vi "Scatter-Gather Write Iterator.vi"(8 "error in (no error)":errorcluster, 9 "Iterations (1000)":i32=110, 10 "Channel Count":i32, 11 "GE 5565PIORC in":refnum<class "GE 5565PIORC Old.lvclass">) -> (0 "error out":errorcluster, 1 "Histogram Graph":T1(graph), 2 "Metrics":T2 {"Transfer Rate" format="%.2pB/s"; "Duration Std. Dev." format="%.0f µs"; "Duration Average" format="%.0f µs"}, 3 "GE 5565PIORC out":refnum<class "GE 5565PIORC Old.lvclass">)   [LabVIEW 2016]
uses:
  Source/GE 5565PIORC/GE 5565PIORC Old.lvclass
  Controls/Throughput Metrics.ctl
  Source/GE 5565PIORC/GE 5565PIORC Old.lvclass/GE 5565PIORC Old.ctl
  Source/GE 5565PIORC/VIs/Block Operations/Allocate Multiple Blocks.vi
  Source/GE 5565PIORC/VIs/DMA/DMA.Create Transfer (Multiple Blocks).vi
  Source/GE 5565PIORC/VIs/Block Operations/Allocate Single Block.vi
  Source/GE 5565PIORC/VIs/DMA/DMA.Transfer Size.vi
  Source/GE 5565PIORC/VIs/Registers/Local Configuration.PCI Address.Set.vi
  Source/GE 5565PIORC/VIs/Registers/Local Configuration.DMADPR0.First Descriptor Address.Set.vi
  Source/GE 5565PIORC/VIs/DMA/DMA.Scatter-Gather.Link Block Descriptors.vi
  Source/GE 5565PIORC/VIs/DMA/DMA.Scatter-Gather.Commit Blocks.vi
  Source/GE 5565PIORC/VIs/Registers/Local Configuration.Local Address.Set.vi
  Source/GE 5565PIORC/VIs/Registers/Local Configuration.Transfer Size.Set.vi
  Source/GE 5565PIORC/VIs/Registers/Local Configuration.DMADPR0.Transfer Direction.Set.vi
  Source/GE 5565PIORC/VIs/Registers/Local Configuration.DMAMODE0.Scatter-Gather Enable.Set.vi
  <vilib>/Utility/error.llb/Clear Errors.vi
  Source/GE 5565PIORC/VIs/Registers/Local Configuration.DMACSR0.DMA Start.Set.vi
  Source/GE 5565PIORC/VIs/Interrupts/Wait for PXI Interrupt Events.vi
  Source/GE 5565PIORC/VIs/Registers/Local Configuration.DMACSR0.DMA Clear Interrupt.Set.vi
  Source/GE 5565PIORC/VIs/Binary Operations/Align to 8-byte Boundary.vi
  Source/GE 5565PIORC/VIs/Binary Operations/Align to 16-byte Boundary.vi
  Source/GE 5565PIORC/VIs/Registers/Local Configuration.Get Register Offset.vi
  Source/GE 5565PIORC/VIs/Binary Operations/Set Bits.vi
  Source/GE 5565PIORC/VIs/Binary Operations/Set Bits U32.vi
  Source/GE 5565PIORC/VIs/Binary Operations/Get Bits.vi
  Source/GE 5565PIORC/VIs/Binary Operations/Get Bits U32.vi
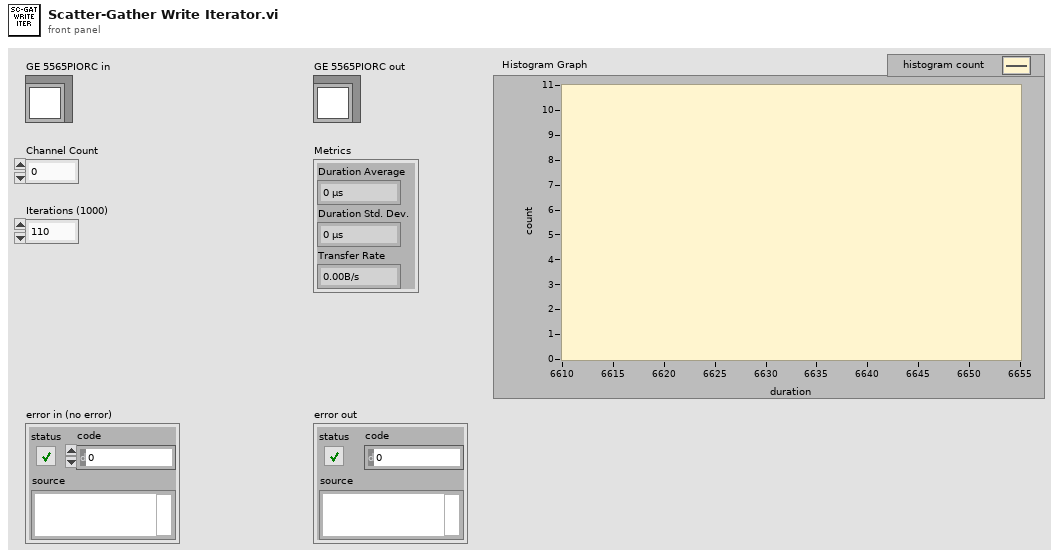
[diagram p1: front panel]
types:
  T1 = cluster{"X Values":dbl[], "Histogram: h(x)":i32[]}
  T2 = typedef "Throughput Metrics.ctl" = cluster{"Duration Average":u32, "Duration Std. Dev.":u32, "Transfer Rate":dbl}
  T3 = typedef "GE 5565PIORC Old.lvclass/DMA Block Descriptor.ctl" = cluster{"descriptor ptr (VISA)":u32, "descriptor size":u32, "descriptor ptr (aligned)":u32, "data ptr (lower)":u32, "data ptr (upper)":u32, "data size":u32, "next descriptor ptr":u32}
  T4 = typedef "GE 5565PIORC Old.lvclass/DMA Transfer Spec.ctl" = cluster{"RFM Address":u32, "Block Descriptors":T3[]}
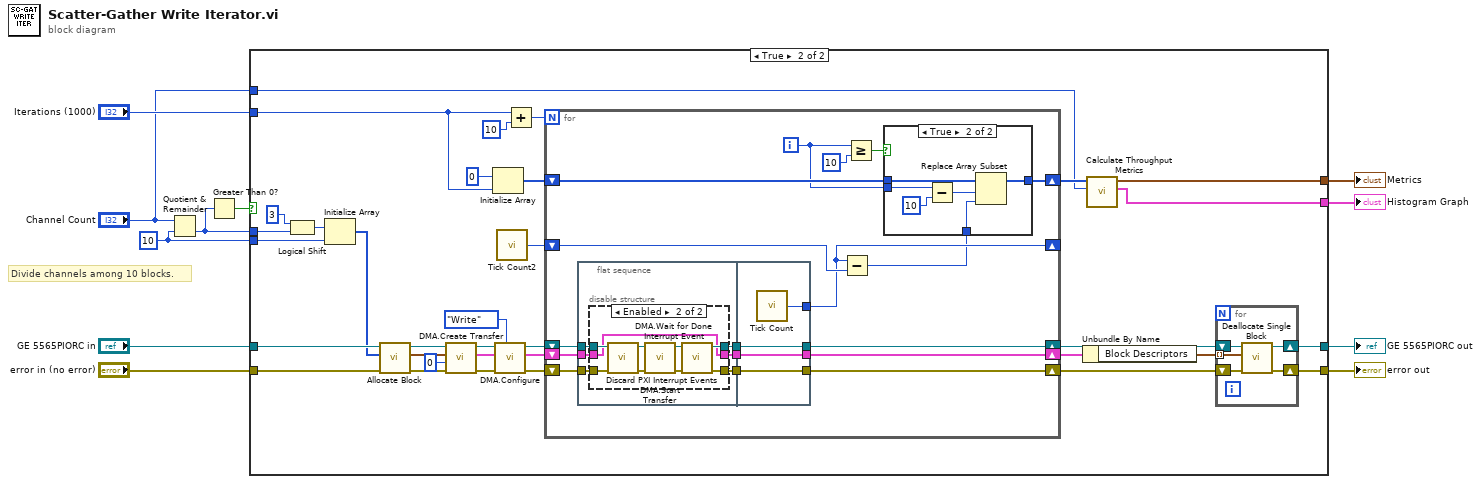
[diagram p0: block diagram]
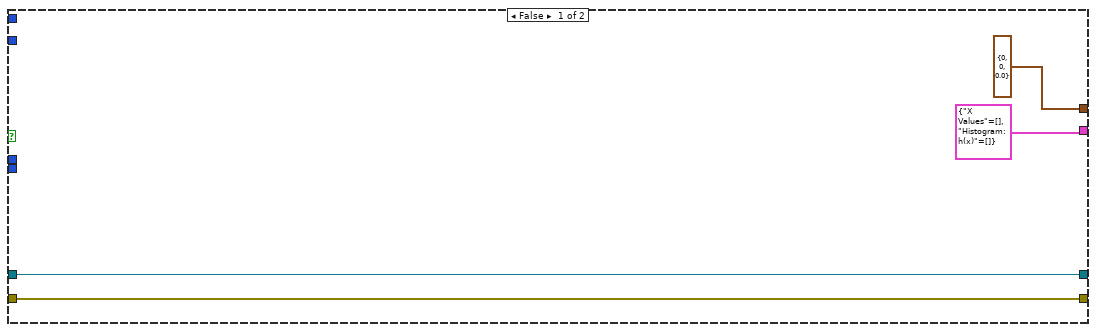
[diagram p2: hidden frame]
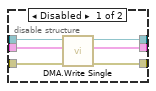
[diagram p4: hidden frame]
diagram:
  w4 = 10 ("y")
  # "Divide channels among 10 blocks."
  n1 = Quotient & Remainder(x="Channel Count", y=w4) -> (floor(x/y)=w2:i32)  [unwired: 1 out]
  n2 = Greater Than 0?(x=w2) -> (x > 0?=w1:bool)
  n3 = case shown="True" w1 {
    tunnel: [w15 w47] -> w11
    tunnel: [w12 w46] -> w10
    tunnel: "Iterations (1000)" -> [_ w40]
    tunnel: [T2 {"Duration Average"=0, "Duration Std. Dev."=0, "Transfer Rate"=0.0} ("Metrics") w36] -> w8
    tunnel: [T1 {"X Values"=[], "Histogram: h(x)"=[]} ("Histogram Graph") w35] -> w7
    tunnel: "GE 5565PIORC in" -> [w12 w34]
    tunnel: "error in (no error)" -> [w15 w33]
    tunnel: w4 -> [_ w29]
    tunnel: w2 -> [_ w28]
    tunnel: "Channel Count" -> [_ w25]
    frame False {
    }
    frame True {
      n4 = Logical Shift(y=i16 3, x=w28) -> (x << y=w27:i32)
      n5 = Initialize Array(w27, w29) -> (w23:i32[])
      n6 = call-poly "Allocate Block.vi"("error in (no error)"=w33, "sizes (bytes)"=w23, "GE 5565PIORC in"=w34) -> ("error out"=w31:errorcluster, "Block Descriptors"=w30:T3[], "GE 5565PIORC out"=w32:refnum<class "GE 5565PIORC Old.lvclass">)  [unwired: 6 in]
      n7 = call-poly "DMA.Create Transfer.vi"("error in (no error)"=w31, "RFM Offset"=u32 0, "Block Descriptors"=w30, "GE 5565PIORC in"=w32) -> ("error out"=w20:errorcluster, "DMA Transfer Spec"=w19:T4, "GE 5565PIORC out"=w21:refnum<class "GE 5565PIORC Old.lvclass">)  [unwired: 4 in, 1 out]
      n8 = Initialize Array(u32 0 ("x-y"), w40) -> (w39:u32[])
      n9 = call "DMA.Configure.vi"("Transfer Direction"=enum16{"Write", "Read"}."Write", "error in (no error)"=w20, "DMA Transfer Spec"=w19, "GE 5565PIORC"=w21) -> ("error out"=w16:errorcluster, "DMA Transfer Spec out"=w17:T4, "GE 5565PIORC out"=w18:refnum<class "GE 5565PIORC Old.lvclass">)  [unwired: 5 in]
      n10 = call "Tick Count2"() -> ("Tick Count(uSec)"=w43:u32)
      n11 = Add(x=w40, y=10) -> (x+y=w49:i32)
      n12 = for {
        N: w49 -> [_]
        shift-right: [w62] -> _
        shift-left: w43 -> [w63]
        shift-right: [w65] -> w44
        shift-left: w18 -> [w71]
        shift-right: [w64] -> w45
        shift-left: w16 -> [w70]
        shift-right: [w60] -> w37
        shift-left: w39 -> [w61]
        shift-right: [w55] -> w26
        shift-left: w17 -> [w69]
        i -> [w58]
        n13 = flat-sequence {
          tunnel: w71 -> [w84]
          tunnel: w70 -> [w83]
          tunnel: w69 -> [w82]
          tunnel: [w80] -> w68
          tunnel: [w79] -> w67
          tunnel: [w81] -> w56
          tunnel: [w103] -> w65
          tunnel: w68 -> [w103]
          tunnel: w67 -> [w102]
          tunnel: [w102] -> w64
          tunnel: [w101] -> w62
          tunnel: w56 -> [w100]
          tunnel: [w100] -> w55
          frame #0 {
            n14 = disable-structure shown="Enabled" {
              disable-tunnel: w84 -> [w90 w97]
              disable-tunnel: w83 -> [w89 w96]
              disable-tunnel: w82 -> [w88 w91]
              disable-tunnel: [w87 w91] -> w81
              disable-tunnel: [w86 w95] -> w80
              disable-tunnel: [w85 w94] -> w79
              frame Disabled {
                n15 = call "DMA.Write Single.vi"("error in (no error)"=w89, "DMA Transfer Spec"=w88, "GE 5565PIORC"=w90) -> ("error out"=w85:errorcluster, "DMA Transfer Spec out"=w87:T4, "GE 5565PIORC out"=w86:refnum<class "GE 5565PIORC Old.lvclass">)  [unwired: 5 in, 1 out]
              }
              frame Enabled {
                n16 = call "Discard PXI Interrupt Events.vi"("error in (no error)"=w96, "GE 5565PIORC in"=w97) -> ("error out"=w99:errorcluster, "GE 5565PIORC out"=w93:refnum<class "GE 5565PIORC Old.lvclass">)  [unwired: 8 in]
                n17 = call "DMA.Start Transfer.vi"("error in (no error)"=w99, "GE 5565PIORC"=w93) -> ("error out"=w98:errorcluster, "GE 5565PIORC out"=w92:refnum<class "GE 5565PIORC Old.lvclass">)  [unwired: 8 in]
                n18 = call "DMA.Wait for Done Interrupt Event.vi"("error in (no error)"=w98, "GE 5565PIORC"=w92) -> ("error out"=w94:errorcluster, "GE 5565PIORC out"=w95:refnum<class "GE 5565PIORC Old.lvclass">)  [unwired: 7 in, 1 out]
              }
            }
          }
          frame #1 {
            n19 = call "Tick Count"() -> ("Tick Count(uSec)"=w101:u32)
          }
        }
        n20 = Subtract(x=w62, y=w63) -> (x-y=w57:u32)
        n21 = Greater Or Equal?(x=w58, y=10) -> (x >= y?=w59:bool)
        n22 = case shown="True" w59 {
          tunnel: w61 -> [w72 w78]
          tunnel: [w72 w77] -> w60
          tunnel: w58 -> [_ w76]
          tunnel: w57 -> [_ w73]
          frame False {
          }
          frame True {
            n23 = Subtract(x=w76, y=10) -> (x-y=w74:i32)
            n24 = Replace Array Subset(array=w78, new element=w73, index=w74) -> (w77:u32[])
          }
        }
      }
      n25 = Unbundle By Name(w26) -> ("Block Descriptors"=w38:T3[])
      n26 = call "Calculate Throughput Metrics.vi"("Channel Count"=w25, "Durations"=w37) -> ("Histogram Graph"=w35:T1, "Metrics"=w36:T2)  [unwired: 8 in]
      n27 = for {
        tunnel: w38 -> [w50] mode=indexing
        shift-right: [w54] -> w47
        shift-left: w45 -> [w52]
        shift-right: [w53] -> w46
        shift-left: w44 -> [w51]
        n28 = call "Deallocate Single Block.vi"("error in (no error)"=w52, "Block Descriptor"=w50, "GE 5565PIORC in"=w51) -> ("error out"=w54:errorcluster, "GE 5565PIORC out"=w53:refnum<class "GE 5565PIORC Old.lvclass">)  [unwired: 7 in]
      }
    }
  }
  "error out" <- w11
  "GE 5565PIORC out" <- w10
  "Metrics" <- w8
  "Histogram Graph" <- w7
